vi "Host Main.vi"() -> ()   [LabVIEW 2017]
doc: "This application launches and executes the Tag Bus Data framework configuration for the specified target alias. This is a simple example of the framework API functions, but may also be a suitable starting point for a Host UI or Thick Client that is running a local version of the framework."
uses:
  <vilib>/NI/Module Execution Interface/Engine Runtime/Execution States.ctl
  <vilib>/NI/Module Execution Interface/Engine Runtime/Fault.ctl
  <vilib>/NI/Tag Bus Module Framework/runtime/error classification.ctl
  <vilib>/NI/Current Value Table/DataTypes/U32_Read.vi
  <vilib>/NI/Current Value Table/DataTypes/Double_Read.vi
  <vilib>/NI/Current Value Table/Type to Enum.vi
  <vilib>/NI/Current Value Table/DataTypes/U32_Type To Enum.vi
  <vilib>/NI/Current Value Table/DataTypes/Double_Type To Enum.vi
  <vilib>/NI/Current Value Table/FGVs/CVT Globals.vi
  <vilib>/NI/Current Value Table/FGVs/Tag Memory.vi
  <vilib>/NI/Current Value Table/Memory Block.vi
  <vilib>/NI/Current Value Table/DataTypes/Double_Memory Block.vi
  <vilib>/NI/Current Value Table/DataTypes/U32_Memory Block.vi
  <vilib>/userdefined/High Color/nirio_resource_hc.ctl
  <vilib>/NI/Module Execution Interface/Engine Runtime/Engine Runtime Interface.lvclass
  <vilib>/NI/DCAF/Tag Editor Core/Framework Configuration Classes/target runtime/PL_Target Runtime.lvclass
  <vilib>/NI/Tag Bus Module Framework/FPGA manager/FPGA manager.lvlib
  <vilib>/rvi/interface/nirviOpenFPGA/nirviOpenFPGA.xnode
  <vilib>/NI/Tag Bus Module Framework/FPGA manager/methods.ctl
  <vilib>/NI/Current Value Table/Current Value Table.lvlib
  <vilib>/NI/Tag Bus Module Framework/runtime/TBM module execution interface.lvclass
panel:
  out "error out":errorcluster
  out "latecount":u32
  in  "Stop Reading Tags":bool=TRUE
  out "duration proc":dbl
  in  "configuration file path":path=path "/home/lvuser/ESM_RT.pcfg"
  in  "target alias":string="cRIO"
  out "engine status":T4(array[cluster])
  in  "stop":bool
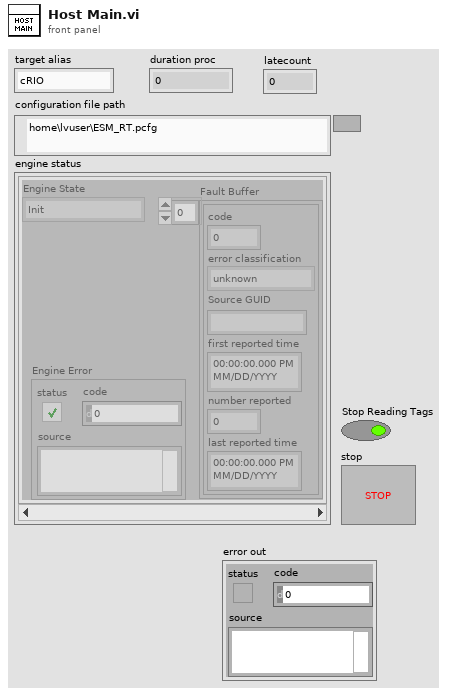
[diagram p1: front panel]
types:
  T1 = typedef "Engine Runtime Interface.lvclass/Execution States.ctl" = enum16{"Init", "Pre-Operational", "Safe-Operational", "Operational", "Stopped"}
  T2 = typedef "Engine Runtime Interface.lvclass/Fault.ctl" = cluster{"code":i32, "error classification":T3, "Source GUID":string, "first reported time":timestamp, "number reported":u32, "last reported time":timestamp}
  T3 = typedef "TBM module execution interface.lvclass/error classification.ctl" = enum16{"unknown", "none", "trivial", "recoverable", "critical"}
  T4 = cluster{"Engine State":T1, "Fault Buffer":T2[], "Engine Error":errorcluster}[]
  T5 = typedef "FPGA manager.lvlib/methods.ctl" = enum16{"initialize bitfile", "cache bitfile", "locate bitfile", "close bitfile", "clear manager"}
  T6 = typedef "nirio_resource_hc.ctl" = tag
  T7 = cluster{"Engine State":T1, "faults":T2[], "Engine Error":errorcluster}
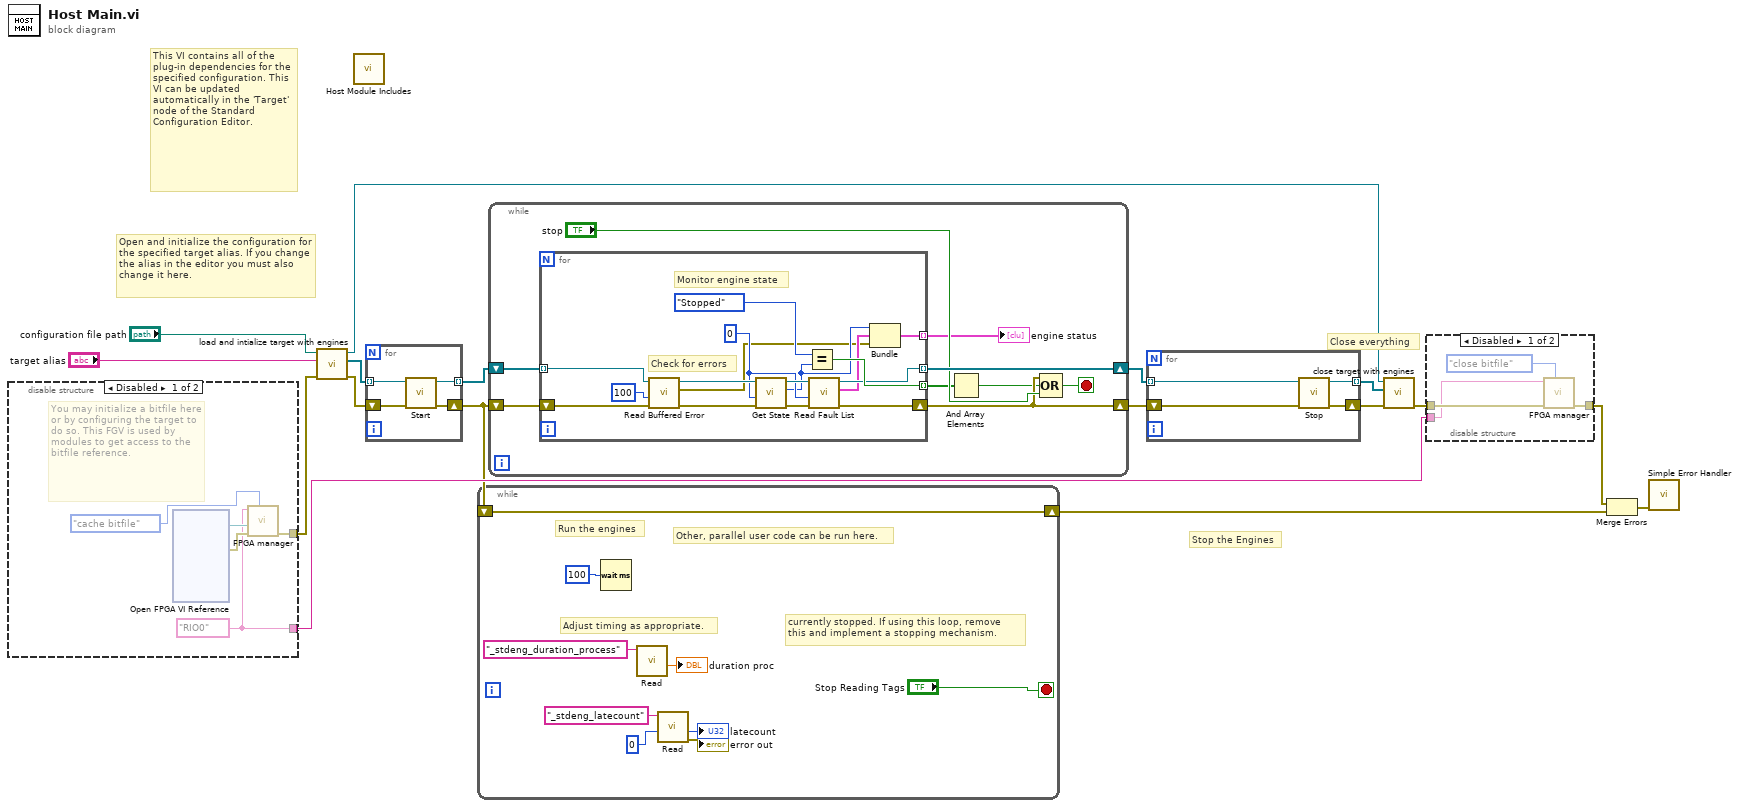
[diagram p0: block diagram]
diagram:
  # "Open and initialize the configuration for the specified target alias. If you change the alias in the editor you must also change it here."
  # "Close everything"
  # "Stop the Engines"
  # "This VI contains all of the plug-in dependencies for the specified configuration. This VI can be updated automatically in the 'Target' node of the Standard Configuration Editor."
  # "Run the engines"
  n1 = disable-structure shown="Disabled" {
    disable-tunnel: [w22 _] -> w7
    disable-tunnel: [w18 _] -> w6
    frame Disabled {
      w18 = T6 "RIO0" ("RIO resource")
      # "You may initialize a bitfile here or by configuring the target to do so. This FGV is used by modules to get access to the bitfile reference."
      n2 = xnode "Open FPGA VI Reference"() -> ("FPGA VI Reference Out"=w20:refnum<k20>, "error out"=w21:errorcluster)  [unwired: 2 in]
      n3 = call <vilib>:"FPGA manager.vi"("action"=methods."cache bitfile", "error in"=w21, "bitfile to cache"=w20, "RIO resource"=w18) -> ("error out"=w22:errorcluster)  [unwired: 5 in, 2 out]
    }
    frame Enabled {
    }
  }
  n4 = call <vilib>:"load and intialize target with engines.vi"("error in"=w7, "target alias"="target alias", "file path"="configuration file path") -> ("error out"=w14:errorcluster, "engine runtime interfaces"=w13:refnum<class "Engine Runtime Interface.lvclass">[], "target runtime"=w10:refnum<class "PL_Target Runtime.lvclass">)  [unwired: 6 in]
  n5 = call "Host Module Includes.vi"() -> ()  [unwired: 12 in]
  n6 = for {
    tunnel: [w26] -> w17 mode=indexing
    tunnel: w13 -> [w23] mode=indexing
    shift-right: [w25] -> w5
    shift-left: w14 -> [w24]
    n7 = call-dynamic "Start.vi"("error in"=w24, "Engine Runtime Interface in"=w23) -> ("error out"=w25:errorcluster, "Engine Runtime Interface out"=w26:refnum<class "Engine Runtime Interface.lvclass">)  [unwired: 8 in]
  }
  n8 = while {
    shift-right: [w33] -> w4
    shift-left: w5 -> [w33]
    stop <- "Stop Reading Tags" stop-if-true
    # "currently stopped. If using this loop, remove \nthis and implement a stopping mechanism."
    # "Adjust timing as appropriate."
    # "Other, parallel user code can be run here."
    n9 = Wait (ms)(milliseconds to wait=u32 100) -> ()  [unwired: 1 out]
    n10 = call-poly <vilib>:"Read.vi"("Tag Name"="_stdeng_duration_process") -> ("Value"=→"duration proc":dbl)  [unwired: 9 in, 1 out]
    n11 = call-poly <vilib>:"Read.vi"("Default"=u32 0, "Tag Name"="_stdeng_latecount") -> ("error out"=→"error out":errorcluster, "Value"=→"latecount":u32)  [unwired: 8 in]
  }
  n12 = while {
    shift-right: [w42] -> w16
    shift-left: w17 -> [w44]
    shift-right: [w39] -> w15
    shift-left: w5 -> [w43]
    stop <- w40 stop-if-true
    n13 = for {
      tunnel: w44 -> [w60] mode=indexing
      tunnel: [w51] -> w42 mode=indexing
      tunnel: [w55] -> w37 mode=indexing
      shift-right: [w50] -> w39
      shift-left: w43 -> [w59]
      tunnel: [w45] -> w38 mode=indexing
      w49 = 0 ("timeout (-1)")
      # "Monitor engine state"
      # "Check for errors"
      n14 = call-dynamic "Read Buffered Error.vi"("error in"=w59, "timeout in ms (0)"=100, "Engine Runtime Interface in"=w60) -> ("error out"=w57:errorcluster, "Engine Error"=w46:errorcluster, "Engine Runtime Interface out"=w58:refnum<class "Engine Runtime Interface.lvclass">)  [unwired: 6 in]
      n15 = call-dynamic "Get State.vi"("error in"=w57, "timeout (-1)"=w49, "Engine Runtime Interface in"=w58) -> ("error out"=w53:errorcluster, "Engine State"=w48:T1, "Engine Runtime Interface out"=w52:refnum<class "Engine Runtime Interface.lvclass">)  [unwired: 6 in]
      n16 = Equal?(x=Execution_States."Stopped" ("Engine State"), y=w48) -> (x = y?=w55:bool)
      n17 = call-dynamic "Read Fault List.vi"("error in"=w53, "timeout (-1)"=w49, "Engine Runtime Interface in"=w52) -> ("error out"=w50:errorcluster, "faults"=w47:T2[], "Engine Runtime Interface out"=w51:refnum<class "Engine Runtime Interface.lvclass">)  [unwired: 6 in]
      n18 = Bundle("Engine State"=w48, "faults"=w47, "Engine Error"=w46) -> (w45:T7)  [unwired: 1 in]
    }
    "engine status" <- w38
    n19 = And Array Elements(Boolean array=w37) -> (logical AND=w36:bool)
    n20 = Compound Arithmetic op=OR(w39, w36, "stop") -> (w40:bool)
  }
  n21 = for {
    tunnel: w16 -> [w64] mode=indexing
    shift-right: [w61] -> w9
    shift-left: w15 -> [w63]
    tunnel: [w62] -> w11 mode=indexing
    n22 = call-dynamic "Stop.vi"("error in"=w63, "Engine Runtime Interface in"=w64) -> ("error out"=w61:errorcluster, "Engine Runtime Interface out"=w62:refnum<class "Engine Runtime Interface.lvclass">)  [unwired: 8 in]
  }
  n23 = call <vilib>:"close target with engines.vi"("error in"=w9, "Engine Runtime Interfaces"=w11, "Target Runtime"=w10) -> ("error out"=w3:errorcluster)  [unwired: 8 in]
  n24 = disable-structure shown="Disabled" {
    disable-tunnel: [w67 w69] -> w2
    disable-tunnel: w3 -> [w68 w69]
    disable-tunnel: w6 -> [w65 _]
    frame Disabled {
      n25 = call <vilib>:"FPGA manager.vi"("action"=methods."close bitfile", "error in"=w68, "RIO resource"=w65) -> ("error out"=w67:errorcluster)  [unwired: 6 in, 2 out]
    }
    frame Enabled {
    }
  }
  n26 = Merge Errors(w2, w4) -> (w1:errorcluster)
  n27 = call <vilib>:"Simple Error Handler.vi"("error in (no error)"=w1) -> ()  [unwired: 4 in, 5 out]
